vi "Permutate String Array.vi"(11 "Array":string[](array[string])) -> (3 "Array":string[][](array[string]))   [LabVIEW 2020]
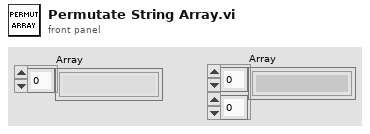
[diagram p1: front panel]
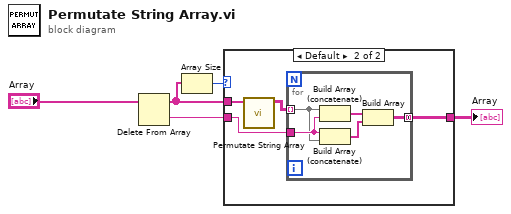
[diagram p0: block diagram]
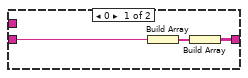
[diagram p2: hidden frame]
diagram:
  n1 = Delete From Array(array="Array") -> (deleted portion=w4:string, array with subset deleted=w2:string[])  [unwired: 2 in]
  n2 = Array Size(array=w2) -> (size(s)=w1:i32)
  n3 = case shown="Default" w1 {
    tunnel: w4 -> [w8 w9]
    tunnel: [w6 w10] -> w3
    tunnel: w2 -> [_ w12]
    frame 0 {
      n4 = Build Array(w8) -> (w7:string[])
      n5 = Build Array(w7) -> (w6:string[][])
    }
    frame Default {
      n6 = call "Permutate String Array.vi"("Array"=w12) -> ("Array"=w11:string[][])  [unwired: 10 in]
      n7 = for {
        tunnel: w11 -> [w14] mode=indexing
        tunnel: [w16] -> w10 mode=concatenating
        tunnel: w9 -> [w15]
        n8 = Build Array (concatenate)(w14, w15) -> (w17:string[])
        n9 = Build Array (concatenate)(w15, w14) -> (w13:string[])
        n10 = Build Array(w17, w13) -> (w16:string[][])
      }
    }
  }
  "Array" <- w3
